vi "Read N Point Positions Velocities.vi"(8 "Error In":errorcluster, 11 "Leap Handle":T1) -> (0 "Error Out":errorcluster, 1 "Point Velocities":cluster{"X":sgl, "Y":sgl, "Z":sgl}[](array[cluster]), 2 "Point Positions":cluster{"X":sgl, "Y":sgl, "Z":sgl}[](array[cluster]), 3 "Leap Handle":T1)   [LabVIEW 2011, in "LVH-Leap.lvlib"]
doc: "<b>Leap Read</b> requests and parses a <b>Frame</b> of data from the Leap Motion Controller. All the data associated with the Frame is organized into a LabVIEW cluster for accessibility.\n\nSpecifics about the data in the Frame cluster can be found by going to <b>Help » Leap Motion Controller Help</b> inside of LabVIEW"
uses:
  LVH-Leap.lvlib
  Private/Type Defs/Leap Handle.ctl
  C:/github/labviewhacker/LVH-Leap/LabVIEW/vi.lib/LabVIEW Hacker/Leap/Private/Libs/LeapCSharp.NET3.5.dll
  Private/Libs/LeapCSharp.NET3.5.dll
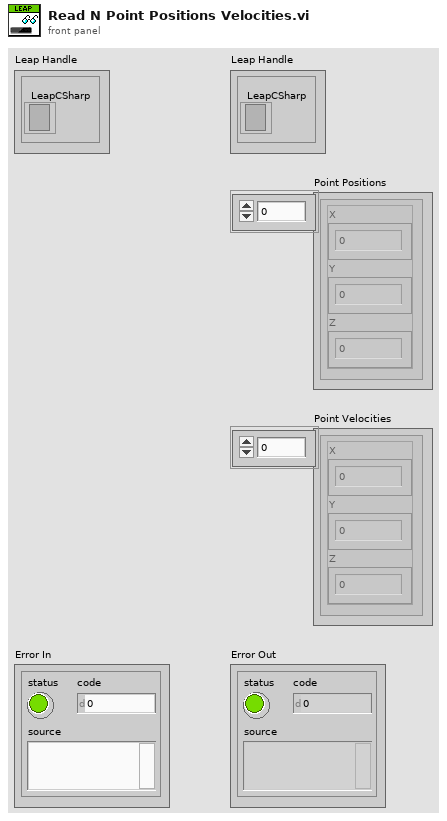
[diagram p1: front panel]
types:
  T1 = typedef "LVH-Leap.lvlib/Leap Handle.ctl" = cluster{"LeapCSharp":refnum<k24>}
  T2 = typedef "LVH-Leap.lvlib/Frame.ctl" = cluster{"ID":i64, "Timestamp":i64, "Current FPS":dbl, "Key Tap Gestures":T3[], "Circle Gestures":T8[], "Screen Tap Gestures":T9[], "Swipe Gestures":T10[], "Hands":T11[]}
  T3 = typedef "LVH-Leap.lvlib/Gesture Key Tap.ctl" = cluster{"Common":T4, "Direction":T7, "Position":T7, "Progress":dbl}
  T4 = typedef "LVH-Leap.lvlib/Gesture Common.ctl" = cluster{"ID":dbl, "Duration (S)":dbl, "Gesture Type":T5, "Gesture State":T6}
  T5 = typedef "LVH-Leap.lvlib/Gesture Type.ctl" = enum16{"Invalid", "Swipe", "Circle", "Screen Tap", "Key Tap"}
  T6 = typedef "LVH-Leap.lvlib/Gesture State.ctl" = enum16{"Invalid", "Start", "Update", "Stop"}
  T7 = typedef "LVH-Leap.lvlib/Vector.ctl" = cluster{"Pitch":sgl, "Yaw":sgl, "Roll":sgl, "Magnitude":sgl, "XYZ":sgl[]}
  T8 = typedef "LVH-Leap.lvlib/Gesture Circle.ctl" = cluster{"Common":T4, "Center":T7, "Normal":T7, "Progress":dbl, "Radius":dbl}
  T9 = typedef "LVH-Leap.lvlib/Gesture Screen Tap.ctl" = cluster{"Common":T4, "Direction":T7, "Position":T7, "Progress":dbl}
  T10 = typedef "LVH-Leap.lvlib/Gesture Swipe.ctl" = cluster{"Common":T4, "Direction":T7, "Position":T7, "Start Position":T7, "Speed":dbl}
  T11 = typedef "LVH-Leap.lvlib/Hand.ctl" = cluster{"Palm Normal":T7, "Palm Position":T7, "Palm Velocity":T7, "Direction":T7, "Palm Position (Stabilized)":T7, "Sphere Center":T7, "Pointables":T12[], "ID":i32, "Time Visible":sgl, "Sphere Radius":sgl}
  T12 = typedef "LVH-Leap.lvlib/Pointable.ctl" = cluster{"Type":T13, "Touch Zone":T14, "ID":i32, "Length":dbl, "Width":dbl, "Time Visible":dbl, "Touch Distance":dbl, "Direction":T7, "Tip Position":T7, "Tip Velocity":T7, "Tip Position (Stabilized)":T7}
  T13 = typedef "LVH-Leap.lvlib/Pointable Type.ctl" = enum16{"Finger", "Tool"}
  T14 = typedef "LVH-Leap.lvlib/Pointable Zone.ctl" = enum16{"None", "Hovering", "Touching"}
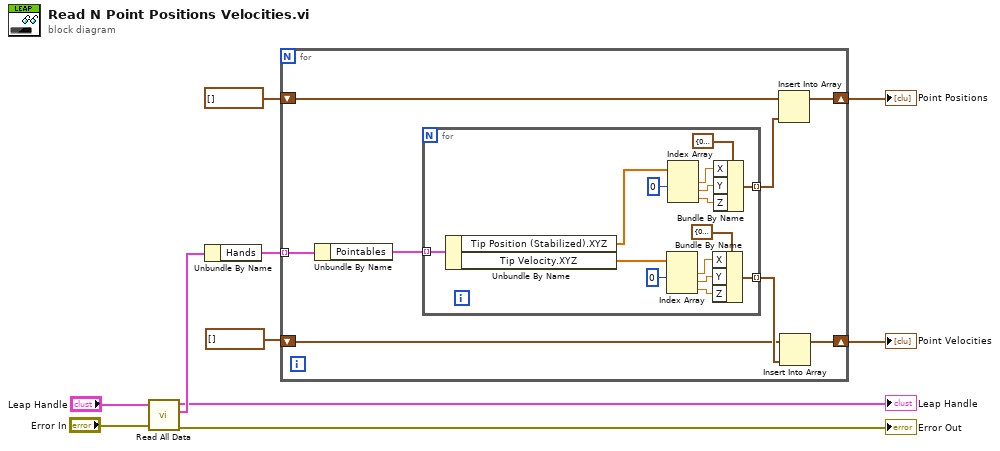
[diagram p0: block diagram]
diagram:
  n1 = call "Read All Data.vi"("Error In"="Error In", "Leap Handle"="Leap Handle") -> ("Error Out"=→"Error Out":errorcluster, "Frame"=w8:T2, "Leap Handle"=→"Leap Handle":T1)  [unwired: 6 in, 1 out]
  n2 = Unbundle By Name(w8) -> ("Hands"=w5:T11[])
  n3 = for {
    tunnel: w5 -> [w18] mode=indexing
    shift-right: [w15] -> w2
    shift-left: cluster{"X":sgl, "Y":sgl, "Z":sgl}[] [] -> [w11]
    shift-right: [w16] -> w1
    shift-left: cluster{"X":sgl, "Y":sgl, "Z":sgl}[] [] -> [w12]
    n4 = Unbundle By Name(w18) -> ("Pointables"=w17:T12[])
    n5 = for {
      tunnel: [w21] -> w14 mode=indexing
      tunnel: [w20] -> w13 mode=indexing
      tunnel: w17 -> [w19] mode=indexing
      n6 = Unbundle By Name(w19) -> ("Tip Position (Stabilized).XYZ"=w32:sgl[], "Tip Velocity.XYZ"=w22:sgl[])
      n7 = Index Array(array=w22, index #1=0 ("index")) -> (element #1=w25:sgl, element #2=w26:sgl, element #3=w27:sgl)  [unwired: 2 in]
      n8 = Index Array(array=w32, index #1=0 ("index")) -> (element #1=w30:sgl, element #2=w29:sgl, element #3=w28:sgl)  [unwired: 2 in]
      n9 = Bundle By Name(cluster=cluster{"X":sgl, "Y":sgl, "Z":sgl} {"X"=0.0, "Y"=0.0, "Z"=0.0}, "X"=w25, "Y"=w26, "Z"=w27) -> (w20:cluster{"X":sgl, "Y":sgl, "Z":sgl})
      n10 = Bundle By Name(cluster=cluster{"X":sgl, "Y":sgl, "Z":sgl} {"X"=0.0, "Y"=0.0, "Z"=0.0}, "X"=w30, "Y"=w29, "Z"=w28) -> (w21:cluster{"X":sgl, "Y":sgl, "Z":sgl})
    }
    n11 = Insert Into Array(array=w11, new element=w14) -> (w15:cluster{"X":sgl, "Y":sgl, "Z":sgl}[])  [unwired: 1 in]
    n12 = Insert Into Array(array=w12, new element=w13) -> (w16:cluster{"X":sgl, "Y":sgl, "Z":sgl}[])  [unwired: 1 in]
  }
  "Point Positions" <- w2
  "Point Velocities" <- w1
